vi "Constructor.vi"(8 "error in (no error)":errorcluster, 11 "Stanford Research PS350 in":refnum<class "Stanford Research PS350.lvclass">) -> (0 "error out":errorcluster, 2 "Init":bool, 3 "Stanford Research PS350 out":refnum<class "Stanford Research PS350.lvclass">)   [LabVIEW 2011, in "Stanford Research PS350.lvclass"]
uses:
  Stanford Research PS350.lvclass
  Stanford Research PS350.lvclass/Stanford Research PS350.ctl
  <instrlib>/Stanford Research PS300 Series/Stanford Research PS300 Series.lvlib
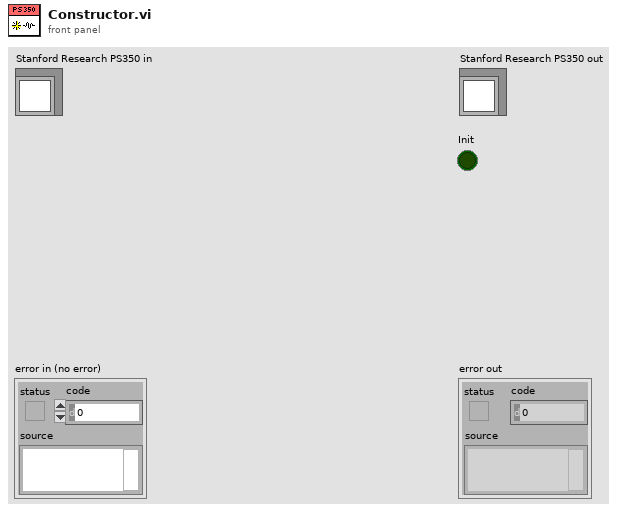
[diagram p1: front panel]
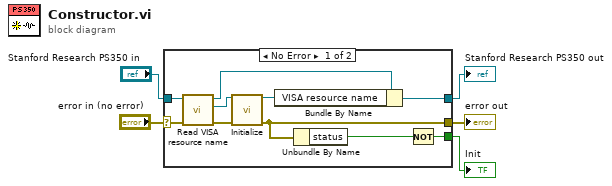
[diagram p0: block diagram]
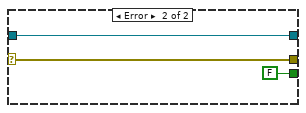
[diagram p2: hidden frame]
diagram:
  n1 = case shown="No Error" "error in (no error)" {
    selector: "error in (no error)" -> [w10 w18]
    tunnel: [w13 w18] -> w4
    tunnel: [w14 w17] -> w2
    tunnel: "Stanford Research PS350 in" -> [w9 w17]
    tunnel: [w12 FALSE ("status")] -> w1
    frame No Error {
      n2 = call-dynamic "Read VISA resource name.vi"("error in (no error)"=w10, "Power Supply in"=w9) -> ("error out"=w6:errorcluster, "VISA resource name"=w7:refnum<visa-resource-name>, "Power Supply out"=w8:refnum<class "Stanford Research PS350.lvclass">)  [unwired: 7 in]
      n3 = call <instrlib>:"Initialize.vi"("VISA resource name"=w7, "error in (no error)"=w6) -> ("VISA resource name out"=w15:refnum<visa-resource-name>, "error out"=w13:errorcluster)  [unwired: 12 in]
      n4 = Bundle By Name(cluster=w8, "VISA resource name"=w15) -> (w14:refnum<class "Stanford Research PS350.lvclass">)
      n5 = Unbundle By Name(w13) -> ("status"=w11:bool)
      n6 = Not(x=w11) -> (.not. x?=w12:bool)
    }
    frame Error {
    }
  }
  "error out" <- w4
  "Stanford Research PS350 out" <- w2
  "Init" <- w1
